vi "Fit_powervsVolts.vi"(8 "error in":errorcluster, 10 "powerdata":dbl[](array[numeric]), 11 "aomdata":dbl[](array[numeric])) -> (0 "error out":errorcluster, 2 "best fit":dynamicdata(graph), 3 "x_out":dbl[](array[numeric]))   [LabVIEW 2016]
panel:
  out "residual":dynamicdata(graph)
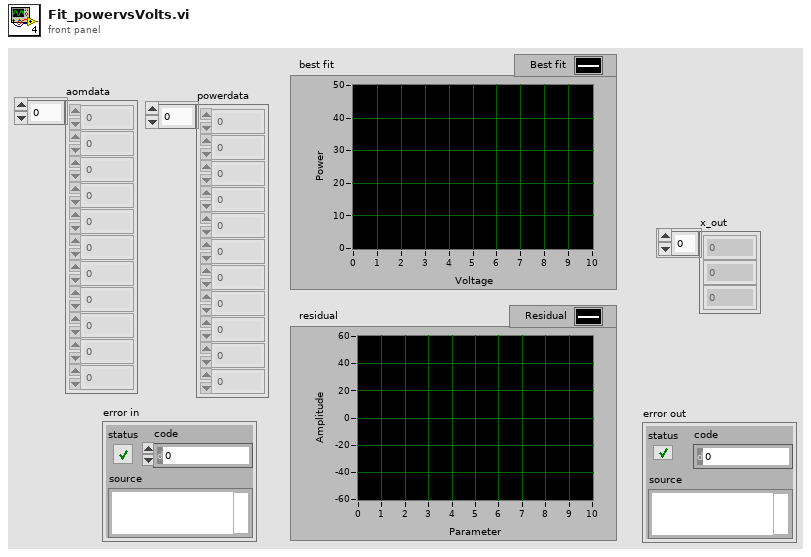
[diagram p1: front panel]
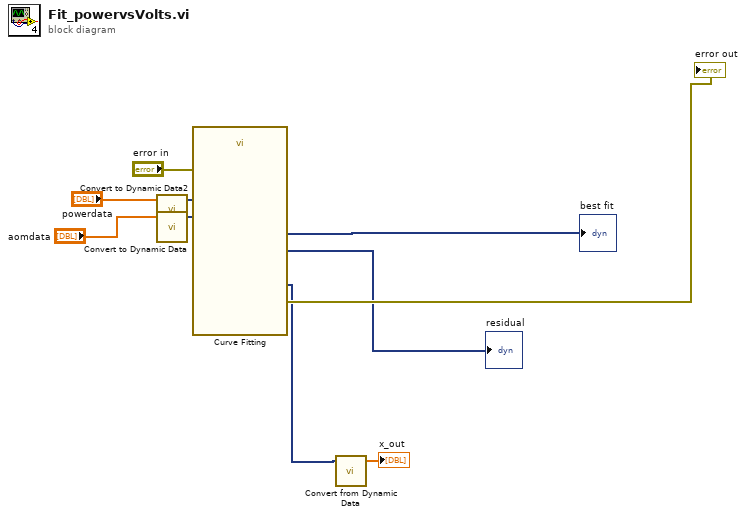
[diagram p0: block diagram]
diagram:
  n1 = call "Convert to Dynamic Data2"("Array"="powerdata") -> ("Dynamic Data Type"=w5:dynamicdata)  [unwired: 3 in]
  n2 = call "Convert to Dynamic Data"("Array"="aomdata") -> ("Dynamic Data Type"=w7:dynamicdata)  [unwired: 3 in]
  n3 = call "Curve Fitting"("error in (no error)"="error in", "Locations"=w7, "Signals"=w5) -> ("error out"=→"error out":errorcluster, "residual"=→"residual":dynamicdata, "best fit"=→"best fit":dynamicdata, "non-linear coefficients"=w2:dynamicdata)  [unwired: 4 in, 1 out]
  n4 = call "Convert from Dynamic Data"("Dynamic Data Type"=w2) -> ("Array"=→"x_out":dbl[])  [unwired: 3 in]
